vi "Untitled 4 (SubVI).vi"(9 "Удалить":bool, 10 "Удаляемый продукт":T1 {"Температура С*" scale=0.0..100.0; "Годен до" format="%<%2d/%2m/%4Y>T"; "Дата изготовления" format="%<%2d/%2m/%4Y>T"}, 11 "Array in":T1[](array[typedef]) {"Температура С*" scale=0.0..100.0; "Годен до" format="%<%2d/%2m/%4Y>T"; "Дата изготовления" format="%<%2d/%2m/%4Y>T"}) -> (1 "String":string, 2 "milliseconds to wait":u32, 3 "Array out":T1[](array[typedef]) {"Температура С*" scale=0.0..100.0; "Годен до" format="%<%2d/%2m/%4Y>T"; "Дата изготовления" format="%<%2d/%2m/%4Y>T"})   [LabVIEW 2020]
uses:
  Control 11.ctl
panel:
  # "Условия хранения"
  # "%"
  # "Пищевая ценность"
  # "Условия хранения"
  # "%"
  # "Пищевая ценность"
  # "Условия хранения"
  # "%"
  # "Пищевая ценность"
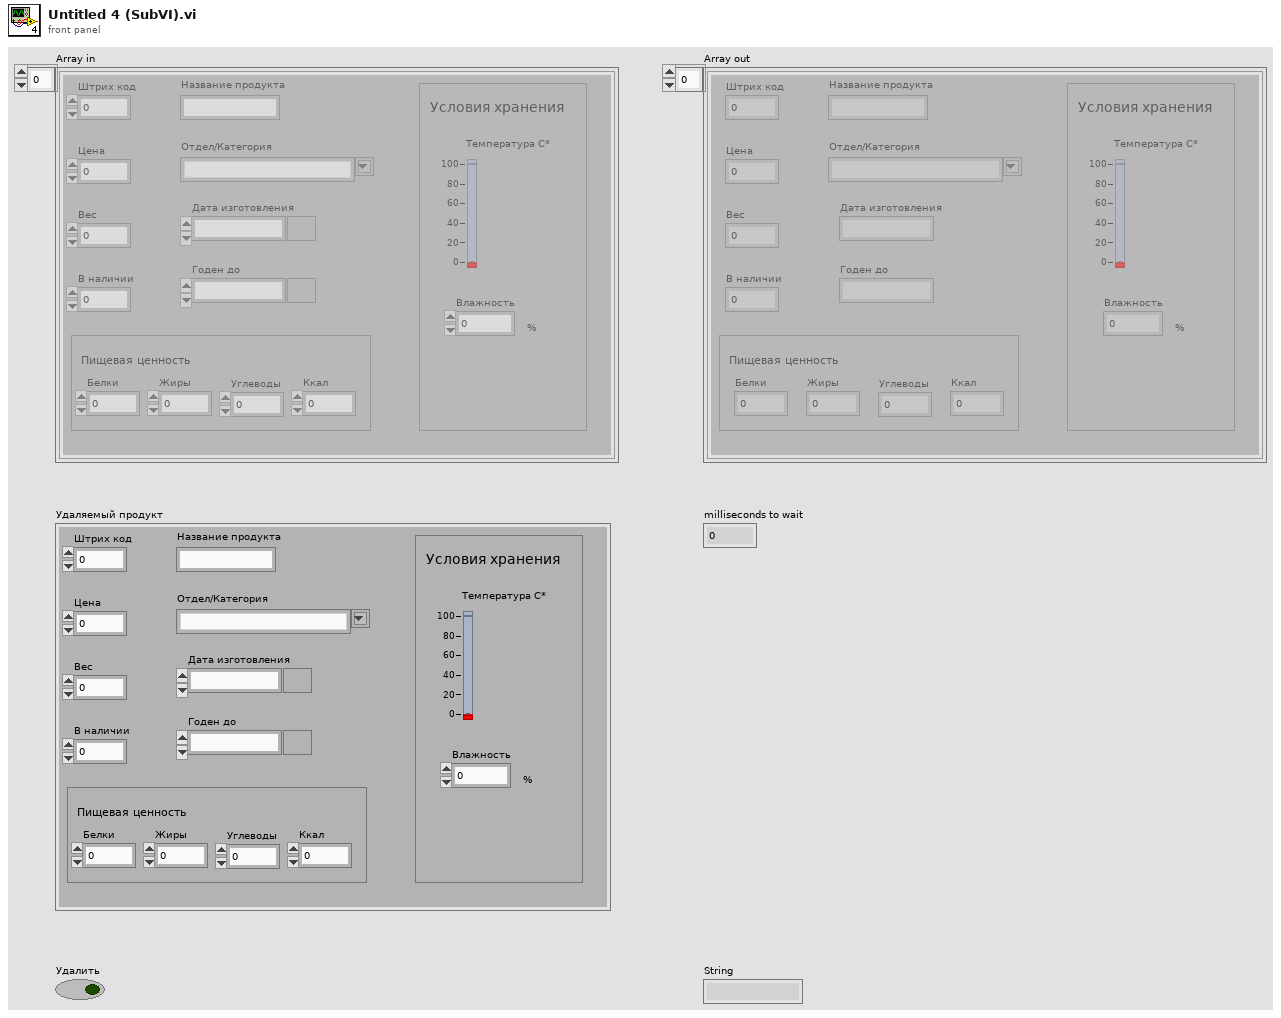
[diagram p1: front panel]
types:
  T1 = typedef "Control 11.ctl" = cluster{"Штрих код":dbl, "Цена":dbl, "Вес":dbl, "В наличии":dbl, "Дата изготовления":timestamp, "Годен до":timestamp, "Название продукта":string, "Температура С*":dbl, "Отдел/Категория":string, "Белки":dbl, "Жиры":dbl, "Углеводы":dbl, "Ккал":dbl, "Влажность":dbl}
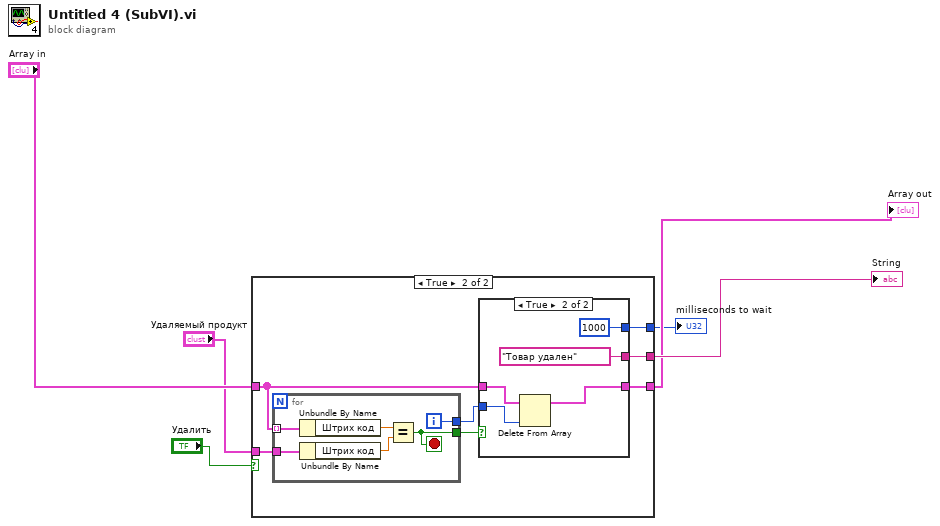
[diagram p0: block diagram]
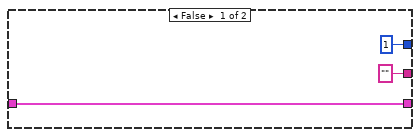
[diagram p2: hidden frame]
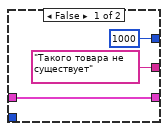
[diagram p3: hidden frame]
diagram:
  n1 = case shown="True" "Удалить" {
    tunnel: ["" w16] -> w6
    tunnel: [u32 1 ("milliseconds to wait") w15] -> w1
    tunnel: "Array in" -> [w7 w14]
    tunnel: "Удаляемый продукт" -> [_ w12]
    tunnel: [w7 w11] -> w5
    frame False {
    }
    frame True {
      n2 = for {
        tunnel: [w21] -> w13
        tunnel: w14 -> [w20] mode=indexing
        tunnel: w12 -> [w19]
        tunnel: [w17] -> w10
        i -> [w17]
        stop <- w21 stop-if-true
        n3 = Unbundle By Name(w20) -> ("Штрих код"=w18:dbl)
        n4 = Unbundle By Name(w19) -> ("Штрих код"=w22:dbl)
        n5 = Equal?(x=w18, y=w22) -> (x = y?=w21:bool)
      }
      n6 = case shown="True" w13 {
        tunnel: ["Такого товара не существует" "Товар удален"] -> w16
        tunnel: [u32 1000 ("milliseconds to wait") u32 1000 ("milliseconds to wait")] -> w15
        tunnel: w14 -> [w23 w29]
        tunnel: [w23 w28] -> w11
        tunnel: w10 -> [_ w30]
        frame False {
        }
        frame True {
          n7 = Delete From Array(array=w29, index=w30) -> (array with subset deleted=w28:T1[])  [unwired: 1 in, 1 out]
        }
      }
    }
  }
  "String" <- w6
  "Array out" <- w5
  "milliseconds to wait" <- w1
